vi "setConfigurationFile.vi"(8 "error in":errorcluster, 9 "content":string, 10 "axis":i32, 11 "connection ID":refnum<k5>) -> (0 "error out":errorcluster, 2 "axis_out":i32, 3 "connection ID":refnum<k5>)   [LabVIEW 2016]
doc: "Load configuration file which either contains JSON parameters or the LUT file itself (as legacy support)"
panel:
  out "params_cluster":cluster{"axis":i32, "content":string}
  in  "Params_cluster":cluster{"integer":i32, "string":string}
  in  "results_cluster":cluster{"errNo":i32}
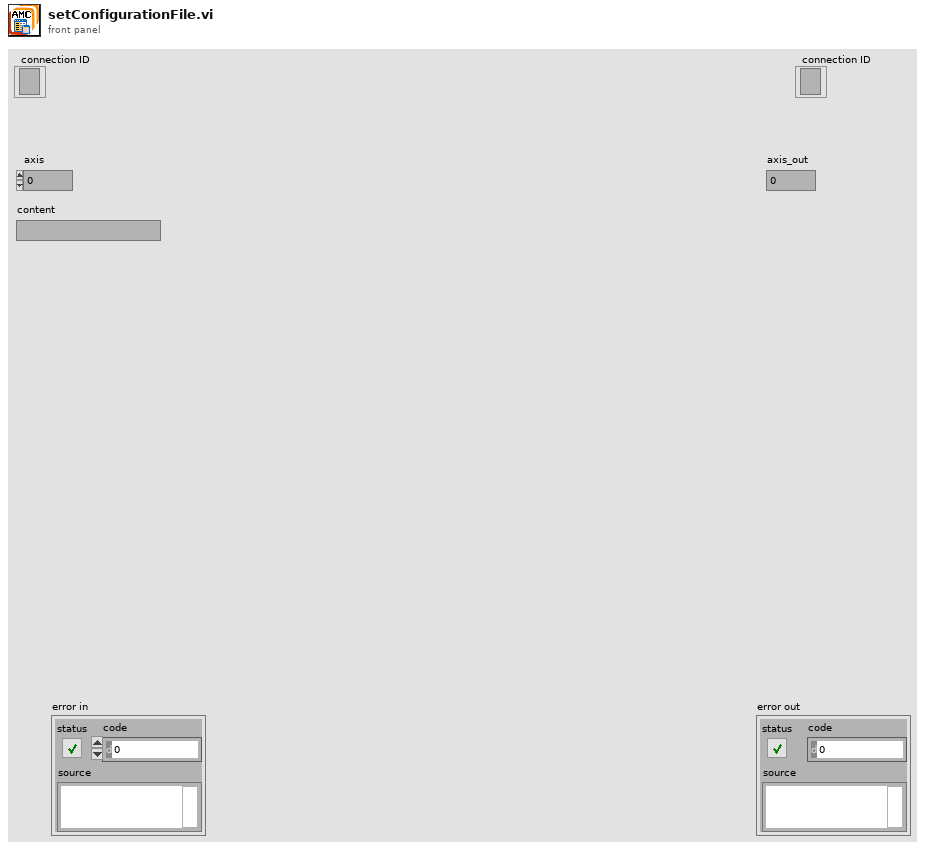
[diagram p1: front panel]
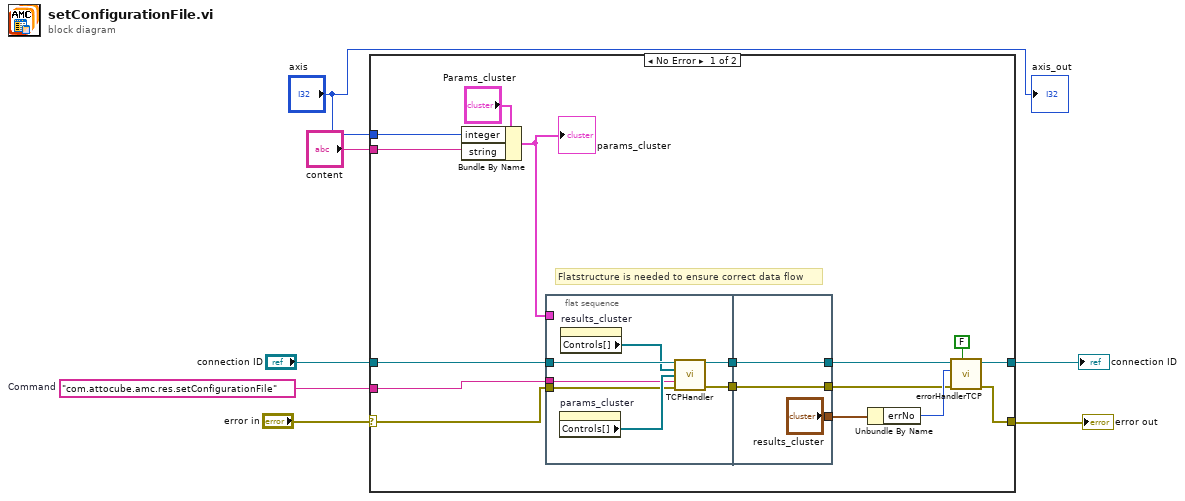
[diagram p0: block diagram]
diagram:
  w3 = "com.attocube.amc.res.setConfigurationFile"  # Command
  n1 = case shown="No Error" "error in" {
    selector: "error in" -> [w8 w35]
    tunnel: [w21 w35] -> w7
    tunnel: [w23 w34] -> w6
    tunnel: "connection ID" -> [w20 w34]
    tunnel: w3 -> [w14 _]
    tunnel: "axis" -> [w10 _]
    tunnel: "content" -> [w9 _]
    frame No Error {
      # "Flatstructure is needed to ensure correct data flow"
      n2 = Bundle By Name(cluster="Params_cluster", "integer"=w10, "string"=w9) -> (w11:cluster{"integer":i32, "string":string})
      "params_cluster" <- w11
      n3 = flat-sequence {
        tunnel: [w29] -> w16
        tunnel: w20 -> [w30]
        tunnel: w14 -> [w26]
        tunnel: [w25] -> w12
        tunnel: w11 -> [_]
        tunnel: w8 -> [w24]
        tunnel: ["results_cluster"] -> w17
        tunnel: [w33] -> w19
        tunnel: w16 -> [w33]
        tunnel: [w31] -> w13
        tunnel: w12 -> [w31]
        frame #0 {
          n4 = property on="params_cluster" class="Clust (strict)"() -> ("Controls[]"=w27:refnum<vi>[])  [unwired: 2 in, 2 out]
          n5 = property on="results_cluster" class="Clust (strict)"() -> ("Controls[]"=w28:refnum<vi>[])  [unwired: 2 in, 2 out]
          n6 = call "TCPHandler.vi"("connection ID"=w30, "results_cluster"=w28, "params_cluster"=w27, "method"=w26, "error"=w24) -> ("connection ID"=w29:refnum<k5>, "error"=w25:errorcluster)  [unwired: 7 in, 2 out]
        }
        frame #1 {
        }
      }
      n7 = Unbundle By Name(w17) -> ("errNo"=w18:i32)
      n8 = call "errorHandlerTCP.vi"("show popup"=FALSE, "error in"=w13, "error number"=w18, "connection ID"=w19) -> ("error out"=w21:errorcluster, "connection ID"=w23:refnum<k5>)  [unwired: 6 in]
    }
    frame Error {
    }
  }
  "error out" <- w7
  "connection ID" <- w6
  "axis_out" <- "axis"
